vi "LDT Parse XML Az El.vi"(8 "error in (no error)":errorcluster, 11 "XML":string="        <hours>12</hours>\n        <minutesTime>10</minutesTime>\n        <secondsTime>35.34</secondsTime>\n") -> (0 "error out":errorcluster, 2 "Elevation":dbl, 3 "Azimuth":dbl)   [LabVIEW 2022 SP3, in "LDT Telescope.lvclass"]
uses:
  LDT Telescope.lvclass
  305062cb-ce46-4c18-a03f-2bcb9346c759.vi
  d3f6fe8a-3317-4632-851b-106c096d98a7.vi
  d981463a-bcb0-4c78-9dc0-0633c0c5472a.vi
  <vilib>/Utility/error.llb/Trim Whitespace.vi
  <vilib>/Utility/error.llb/Trim Whitespace One-Sided.vi
  Telescope.lvclass
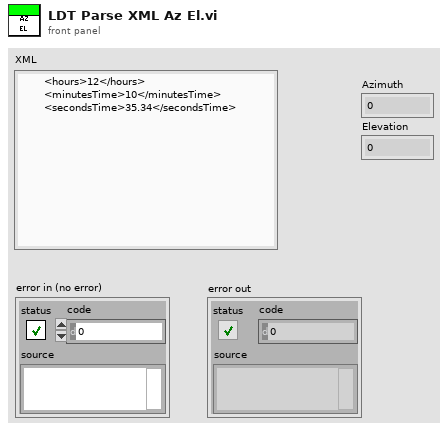
[diagram p1: front panel]
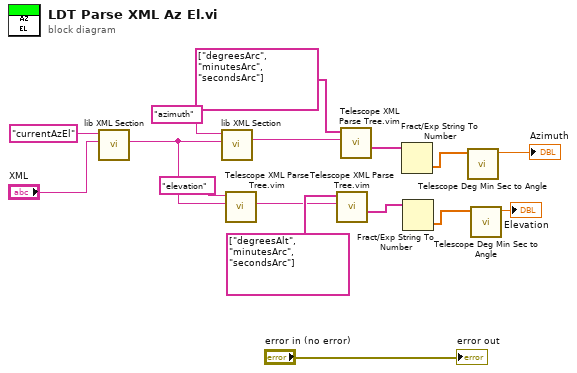
[diagram p0: block diagram]
diagram:
  n1 = call "lib XML Section.vi"("XML String"="XML", "XML Topic"="currentAzEl") -> ("XML Topic Body"=w9:string)  [unwired: 7 in, 2 out]
  n2 = call "lib XML Section.vi"("XML String"=w9, "XML Topic"="azimuth") -> ("XML Topic Body"=w15:string)  [unwired: 7 in, 2 out]
  n3 = call "Telescope XML Parse Tree.vim"("XML String"=w9, "XML Topic"="elevation") -> ("XML Topic Body"=w6:string)  [unwired: 6 in, 3 out]
  n4 = call "Telescope XML Parse Tree.vim"("XML String"=w6, "XML Topic"=string[] ["degreesAlt", "minutesArc", "secondsArc"]) -> ("Body"=w5:string[])  [unwired: 6 in, 3 out]
  n5 = call "Telescope XML Parse Tree.vim"("XML String"=w15, "XML Topic"=string[] ["degreesArc", "minutesArc", "secondsArc"]) -> ("Body"=w12:string[])  [unwired: 6 in, 3 out]
  n6 = Fract/Exp String To Number(string=w12) -> (number=w4:dbl[])  [unwired: 3 in, 1 out]
  n7 = Fract/Exp String To Number(string=w5) -> (number=w3:dbl[])  [unwired: 3 in, 1 out]
  n8 = call "Telescope Deg Min Sec to Angle.vi"("deg min sec"=w4) -> ("result"=→"Azimuth":dbl)  [unwired: 10 in]
  n9 = call "Telescope Deg Min Sec to Angle.vi"("deg min sec"=w3) -> ("result"=→"Elevation":dbl)  [unwired: 10 in]
  "error out" <- "error in (no error)"
